vi "Subtract.vi"(10 "x":dbl, 11 "y":dbl) -> (2 "x-y":dbl)   [LabVIEW 2021]
panel:
  in  "Slide":dbl(slide) scale=0.0..10.0
  in  "stop":bool
  # "MORE CHANGES"
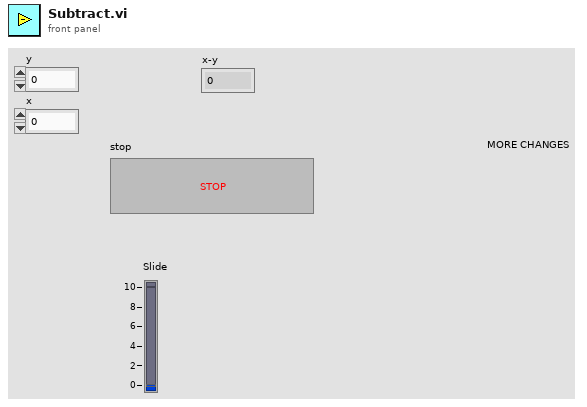
[diagram p1: front panel]
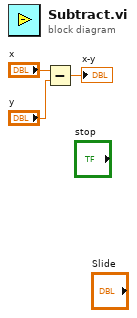
[diagram p0: block diagram]
diagram:
  n1 = Subtract(x="x", y="y") -> (x-y=→"x-y":dbl)
